vi "Jenkins - Call Build.vi"(8 "error in (no error)":errorcluster, 9 "Parameters":variant, 10 "Script Job Name (Within Build Script Folder)":string, 11 "IP Address":string) -> (0 "error out":errorcluster)   [LabVIEW 2014]
uses:
  <vilib>/httpClient/LabVIEWHTTPClient.lvlib
  <vilib>/wsapi/NI_WebServices.lvlib
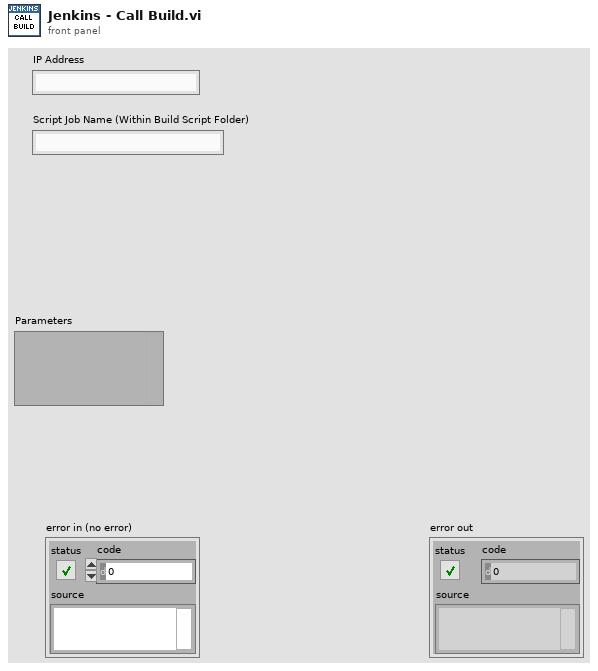
[diagram p1: front panel]
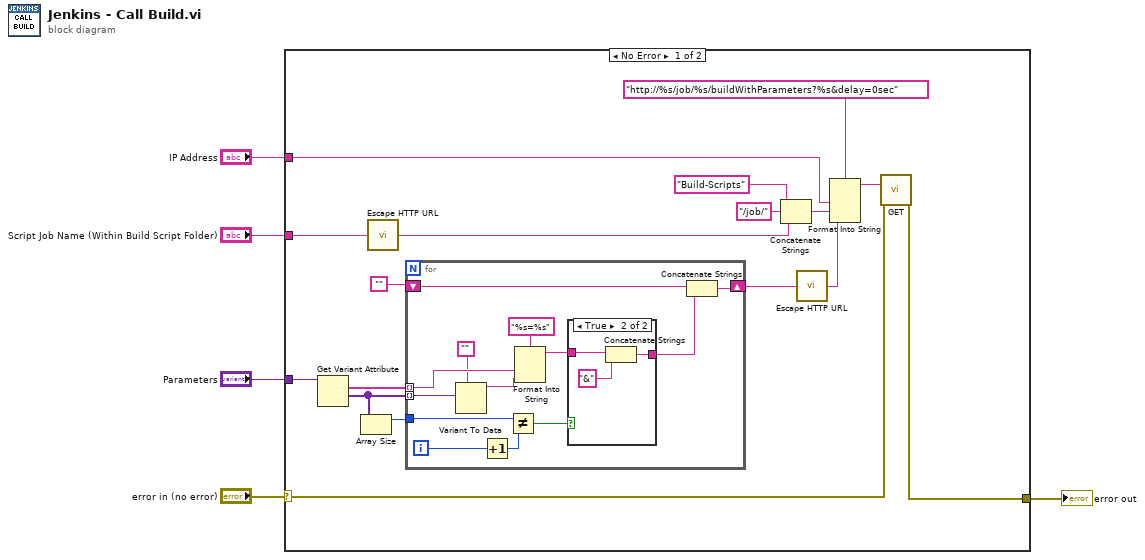
[diagram p0: block diagram]
diagram:
  n1 = case shown="No Error" "error in (no error)" {
    selector: "error in (no error)" -> [w11 w40]
    tunnel: "Script Job Name (Within Build Script Folder)" -> [w10 _]
    tunnel: "IP Address" -> [w18 _]
    tunnel: [w17 w40] -> w3
    tunnel: "Parameters" -> [w8 _]
    frame No Error {
      n2 = Get Variant Attribute(Variant=w8) -> (names=w7:string[], values=w6:variant[])  [unwired: 3 in, 2 out]
      n3 = Array Size(array=w6) -> (size(s)=w15:i32)
      n4 = call <vilib>:"Escape HTTP URL.vi"("unescaped string in"=w10) -> ("escaped string out"=w9:string)
      n5 = for {
        shift-right: [w33] -> w14
        shift-left: "" -> [w34]
        tunnel: w15 -> [w30]
        tunnel: w7 -> [w26] mode=indexing
        tunnel: w6 -> [w25] mode=indexing
        i -> [w32]
        n6 = Variant To Data(type="", Variant=w25) -> (data=w23:string)  [unwired: 1 in, 1 out]
        n7 = Increment(x=w32) -> (x+1=w31:i32)
        n8 = Not Equal?(x=w30, y=w31) -> (x != y?=w29:bool)
        n9 = Format Into String(format string="%s=%s", w26, w23) -> (resulting string=w28:string)  [unwired: 2 in, 1 out]
        n10 = case shown="True" w29 {
          tunnel: w28 -> [w36 w39]
          tunnel: [w36 w37] -> w27
          frame False {
          }
          frame True {
            n11 = Concatenate Strings(w39, "&" ("string")) -> (w37:string)
          }
        }
        n12 = Concatenate Strings(w34, w27) -> (w33:string)
      }
      n13 = Concatenate Strings("Build-Scripts" ("JSON"), "/job/" ("string"), w9) -> (w19:string)
      n14 = call <vilib>:"Escape HTTP URL.vi"("unescaped string in"=w14) -> ("escaped string out"=w13:string)
      n15 = Format Into String(format string="http://%s/job/%s/buildWithParameters?%s&delay=0sec", w18, w19, w13) -> (resulting string=w22:string)  [unwired: 2 in, 1 out]
      n16 = call <vilib>:"GET.vi"("url"=w22, "error in (no error)"=w11) -> ("error out"=w17:errorcluster)  [unwired: 10 in, 3 out]
    }
    frame Error {
    }
  }
  "error out" <- w3
